vi "Default Motor Parameters.vi"() -> ()   [LabVIEW 2014]
uses:
  EMC API/EMC_Typedef_Motor_Parameters.ctl
panel:
  in  "Default Motor Parameters":T1={"position"=10000.0, "velocity"=10000.0, "acceleration"=100000.0, "deceleration"=100000.0, "accel. jerk"=1000000.0, "decel. jerk"=1000000.0}
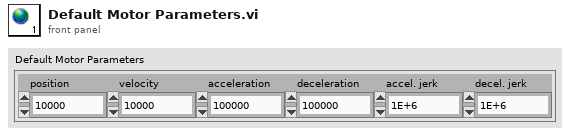
[diagram p1: front panel]
types:
  T1 = typedef "EMC_Typedef_Motor_Parameters.ctl" = cluster{"position":dbl, "velocity":dbl, "acceleration":dbl, "deceleration":dbl, "accel. jerk":dbl, "decel. jerk":dbl}
diagram:
